vi "Write Self Attributes.vi"(10 "Self Attributes":refnum<class "Attributes.lvclass">, 11 "Core Actor in":refnum<class "Core Actor.lvclass">) -> (3 "Core Actor out":refnum<class "Core Actor.lvclass">)   [LabVIEW 2025, in "jettl.lvlib" / "Base Actor.lvlib" / "Core Actor.lvclass"]
uses:
  Core Actor.lvclass
  Attributes/Attributes.lvclass
  Core Actor.lvclass/Core Actor.ctl
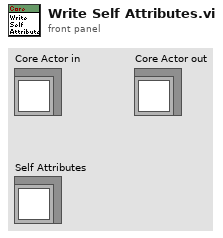
[diagram p1: front panel]
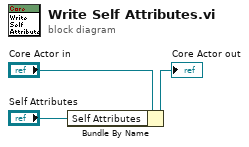
[diagram p0: block diagram]
diagram:
  n1 = Bundle By Name(cluster="Core Actor in", "Self Attributes"="Self Attributes") -> (→"Core Actor out":refnum<class "Core Actor.lvclass">)
